vi "Vision Research Phantom Series PhMemorySize.vi"(0 "CN in":u32=1, 5 "Error In (no error)":errorcluster) -> (14 "CN out":u32=1, 15 "pDRAM":u32, 17 "pNVMSize":u32, 19 "Error Out":errorcluster)   [LabVIEW 2013, in "VRI.lvlib"]
doc: "PhCon dll\n\nPhMemorySize\nHRESULT PhMemorySize (UINT CN, PUINT pDRAMSize, PUINT pNVMSize);\n\nParameters Description\nCN (in) Camera number\npDRAMSize (out) The DRAM memory size in MB\npNVMSize (out) The NonVolatile memory size in MB\nReturn HRESULT (0=Ok)\nComments Provide the size of the camera DRAM and NonVolatileMemory\n\nWritten by:\nBLOOMY CONTROLS, INC\nWINDSOR, CT 06095, USA\n860-298-9925\nwww.bloomy.com\nV1.0.0\nMay, 2004"
uses:
  VRI.lvlib
  Phantom DLLs/PhCon.dll
panel:
  # "For instructions on the use of this VI, press Ctrl+H to display the help window and move the mouse over the icon, controls, and indicators"
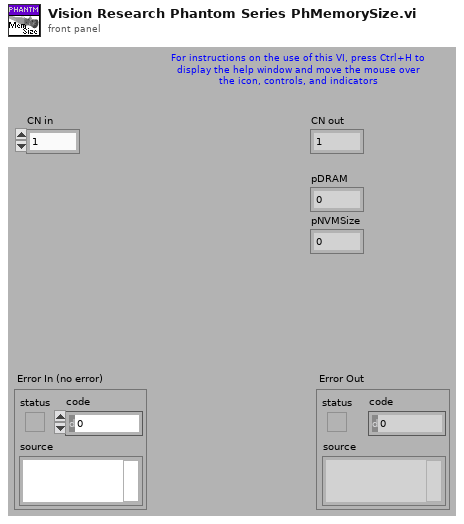
[diagram p1: front panel]
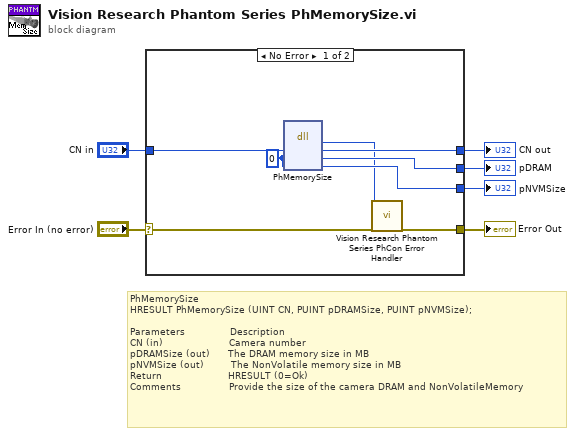
[diagram p0: block diagram]
diagram:
  # "PhMemorySize\nHRESULT PhMemorySize (UINT CN, PUINT pDRAMSize, PUINT pNVMSize);\n\nParameters               Description\nCN (in)                      Camera number\npDRAMSize (out)      The DRAM memory size in MB\npNVMSize (out)         The NonVolatile memory size in MB\nReturn                      HRESULT (0=Ok)\nComments                Provide the size of the camera DRAM and NonVolatileMemory"
  n1 = case shown="No Error" "Error In (no error)" {
    selector: "Error In (no error)" -> [w14 w16]
    tunnel: [w13 w16] -> w5
    tunnel: "CN in" -> [w12 w15]
    tunnel: [w11 w15] -> w3
    tunnel: [w10 _] -> w2
    tunnel: [w9 _] -> w1
    frame No Error {
      w7 = u32 0 ("pDRAM")
      n2 = dll-call lib="C:/Projects/SDK/32-bit/Vision Research Phantom Series Labview Driver/Phantom DLLs/PhCon.dll" fn="PhMemorySize"("CN"=w12, "pDRAM"=w7, "pNVMSize"=w7) -> ("HRESULT"=w8:i32, "CN"=w11:u32, "pDRAM"=w10:u32, "pNVMSize"=w9:u32)  [unwired: 3 in, 2 out]
      n3 = call "Vision Research Phantom Series PhCon Error Handler.vi"("ErrNo"=w8, "Error In (no error)"=w14) -> ("Error Out"=w13:errorcluster)  [unwired: 17 out]
    }
    frame Error {
    }
  }
  "Error Out" <- w5
  "CN out" <- w3
  "pDRAM" <- w2
  "pNVMSize" <- w1
